vi "GetSensorGroupById.vi"(10 "sensor group id":string, 11 "asset nodes in":T5[](array[typedef])) -> (1 "found":bool, 2 "sensor group":T1, 3 "asset nodes out":T5[](array[typedef]))   [LabVIEW 2017, in "DeviceModelHelpers.lvlib"]
uses:
  <vilib>/addons/InsightCM/Utilities/DeviceModelHelpers/DeviceModelHelpers.lvlib
  <vilib>/addons/InsightCM/MessageBus/Base/controls/AssetNode.ctl
  <vilib>/addons/InsightCM/MessageBus/Base/controls/AssetState.ctl
  <vilib>/addons/InsightCM/MessageBus/Base/controls/KeyValuePair.ctl
  <vilib>/addons/InsightCM/MessageBus/Base/controls/AssetNodeSensorGroup.ctl
  <vilib>/addons/InsightCM/MessageBus/Base/controls/WirelessCollectionConfig.ctl
  <vilib>/addons/InsightCM/MessageBus/Base/controls/Condition.ctl
  <vilib>/addons/InsightCM/MessageBus/Base/controls/OperatingState.ctl
  <vilib>/addons/InsightCM/MessageBus/Base/controls/Trigger.ctl
  <vilib>/addons/InsightCM/MessageBus/Base/controls/Metric.ctl
  <vilib>/addons/InsightCM/MessageBus/Base/controls/TrendAlarmRule.ctl
  <vilib>/addons/InsightCM/MessageBus/Base/controls/TrendAlarmLevel.ctl
  <vilib>/addons/InsightCM/MessageBus/Base/controls/AlarmAction.ctl
  <vilib>/addons/InsightCM/MessageBus/Base/controls/AssetNodeReference.ctl
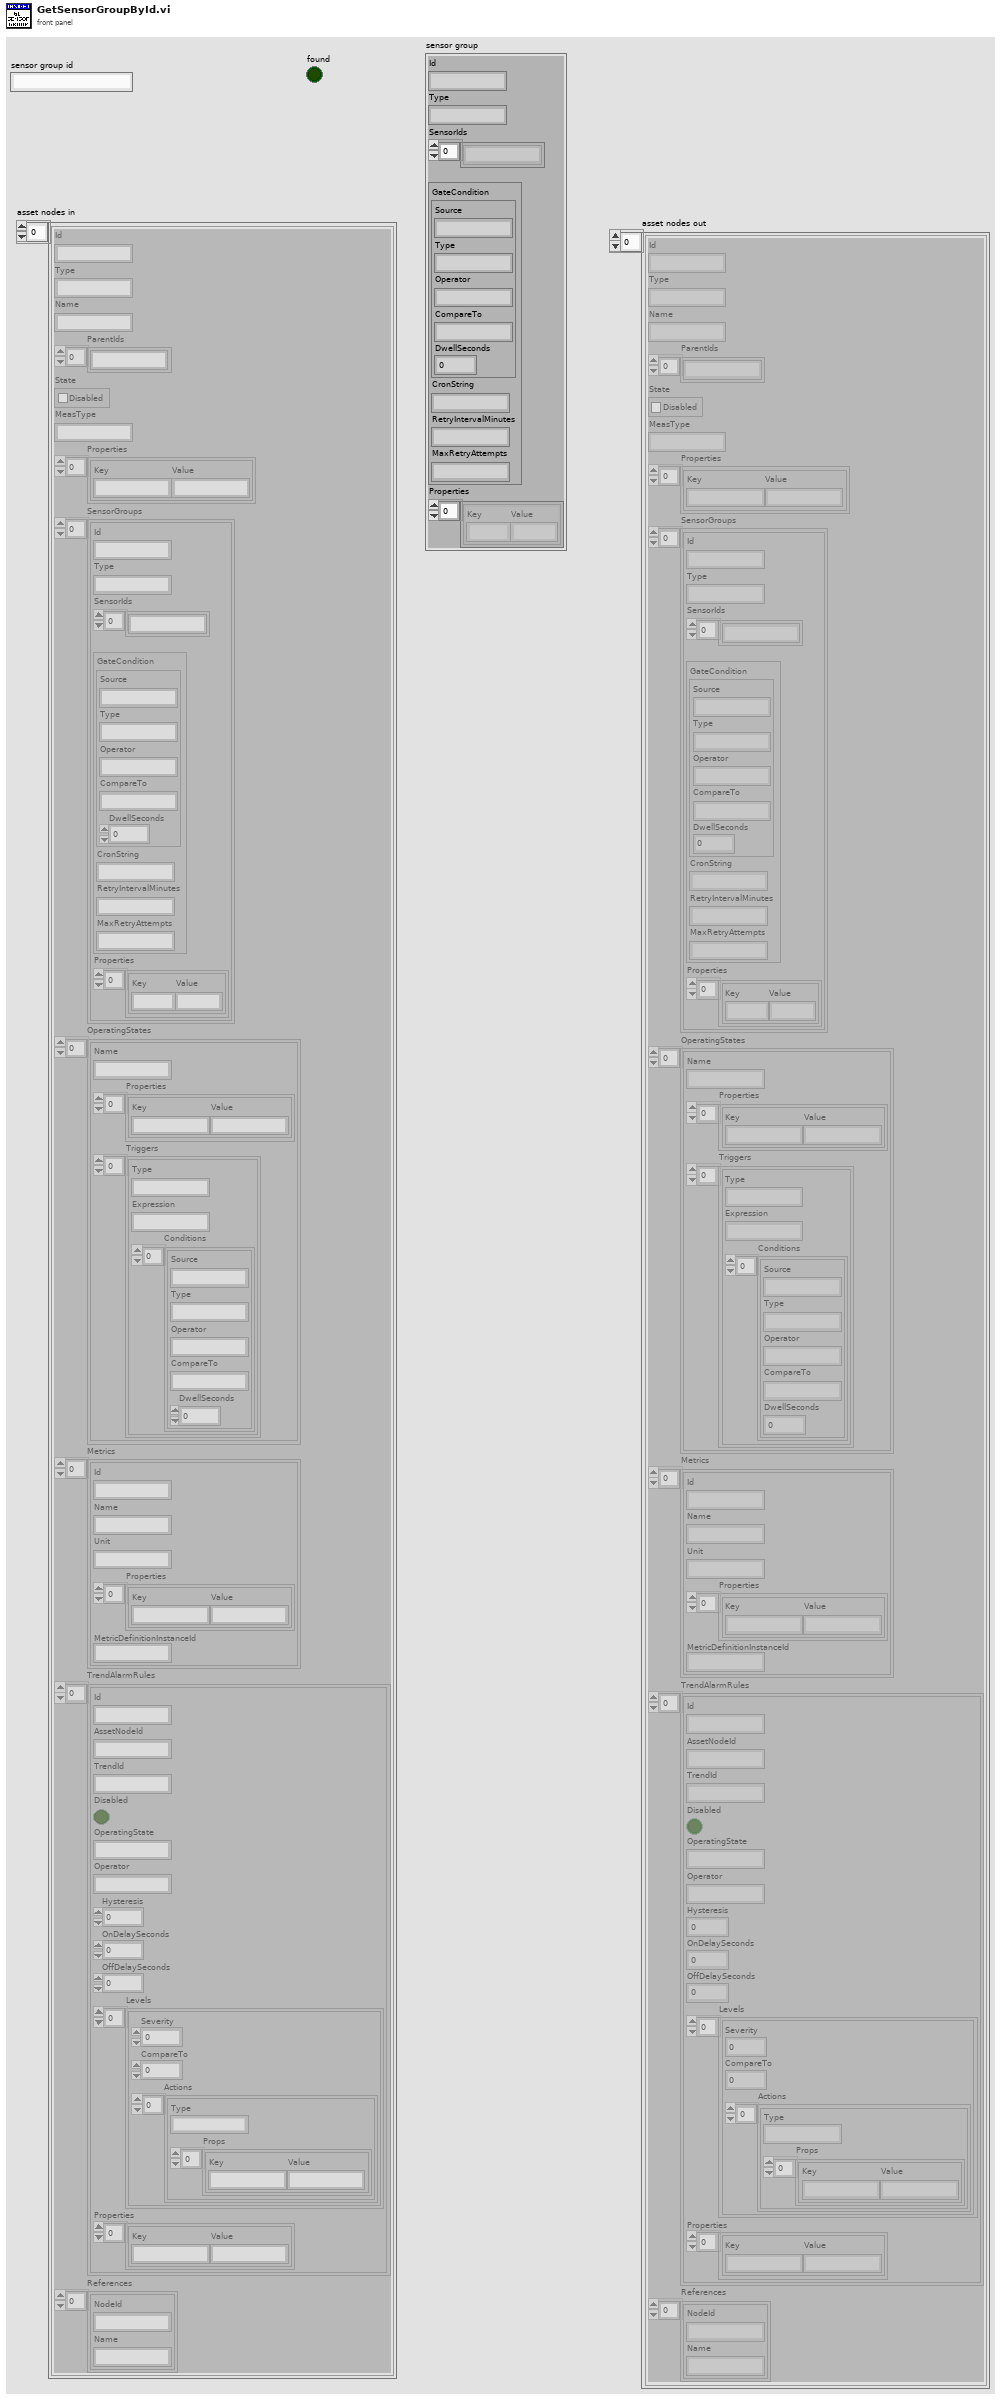
[diagram p1: front panel]
types:
  T1 = typedef "AssetNodeSensorGroup.ctl" = cluster{"Id":string, "Type":string, "SensorIds":string[], "CollectionConfig":T2, "Properties":T4[]}
  T2 = typedef "WirelessCollectionConfig.ctl" = cluster{"GateCondition":T3, "CronString":string, "RetryIntervalMinutes":string, "MaxRetryAttempts":string}
  T3 = typedef "Condition.ctl" = cluster{"Source":string, "Type":string, "Operator":string, "CompareTo":string, "DwellSeconds":dbl}
  T4 = typedef "KeyValuePair.ctl" = cluster{"Key":string, "Value":string}
  T5 = typedef "AssetNode.ctl" = cluster{"Id":string, "Type":string, "Name":string, "ParentIds":string[], "State":T6, "MeasType":string, "Properties":T4[], "SensorGroups":T1[], "OperatingStates":T7[], "Metrics":T9[], "TrendAlarmRules":T10[], "References":T13[]}
  T6 = typedef "AssetState.ctl" = cluster{"Disabled":bool}
  T7 = typedef "OperatingState.ctl" = cluster{"Name":string, "Properties":T4[], "Triggers":T8[]}
  T8 = typedef "Trigger.ctl" = cluster{"Type":string, "Expression":string, "Conditions":T3[]}
  T9 = typedef "Metric.ctl" = cluster{"Id":string, "Name":string, "Unit":string, "Properties":T4[], "MetricDefinitionInstanceId":string}
  T10 = typedef "TrendAlarmRule.ctl" = cluster{"Id":string, "AssetNodeId":string, "TrendId":string, "Disabled":bool, "OperatingState":string, "Operator":string, "Hysteresis":dbl, "OnDelaySeconds":dbl, "OffDelaySeconds":dbl, "Levels":T11[], "Properties":T4[]}
  T11 = typedef "TrendAlarmLevel.ctl" = cluster{"Severity":i32, "CompareTo":dbl, "Actions":T12[]}
  T12 = typedef "AlarmAction.ctl" = cluster{"Type":string, "Props":T4[]}
  T13 = typedef "AssetNodeReference.ctl" = cluster{"NodeId":string, "Name":string}
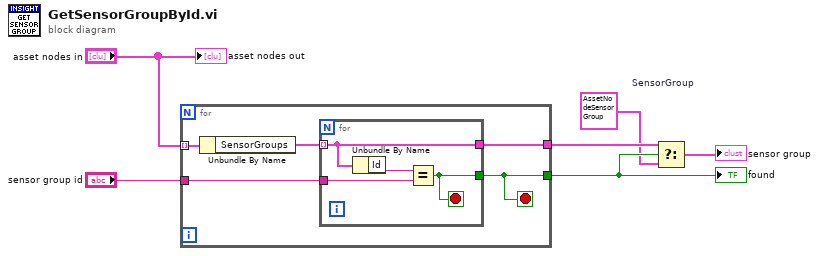
[diagram p0: block diagram]
diagram:
  w2 = T1 {"Id"="", "Type"="", "SensorIds"=[], "CollectionConfig"={"GateCondition"={"Source"="", "Type"="", "Operator"="", "CompareTo"="", "DwellSeconds"=0.0}, "CronString"="", "RetryIntervalMinutes"="", "MaxRetryAttempts"=""}, "Properties"=[]}  # SensorGroup
  n1 = for {
    tunnel: "asset nodes in" -> [w9] mode=indexing
    tunnel: "sensor group id" -> [w10]
    tunnel: [w8] -> w4
    tunnel: [w7] -> w5
    stop <- w7 stop-if-true
    n2 = Unbundle By Name(w9) -> ("SensorGroups"=w11:T1[])
    n3 = for {
      tunnel: w11 -> [w15] mode=indexing
      tunnel: w10 -> [w13]
      tunnel: [w15] -> w8
      tunnel: [w12] -> w7
      stop <- w12 stop-if-true
      n4 = Unbundle By Name(w15) -> ("Id"=w14:string)
      n5 = Equal?(x=w14, y=w13) -> (x = y?=w12:bool)
    }
  }
  "found" <- w5
  n6 = Select(t=w4, s=w5, f=w2) -> (s? t:f=→"sensor group":T1)
  "asset nodes out" <- "asset nodes in"
